vi "Lockin-4461_Multiple Inputs and Outputs_KH_functional_global.vi"(8 "stop":bool) -> ()   [LabVIEW 2013]
uses:
  <vilib>/Analysis/4window.llb/windowTd.ctl
  <vilib>/Analysis/baseanly.llb/Mean (DBL).vi
  <vilib>/Analysis/2dsp.llb/Decimate (single shot, DBL).vi
  <vilib>/DAQmx/write.llb/DAQmx Write (Analog 1D Wfm NChan NSamp).vi
  DAQ-Lockin-SubVI/Lock-in Globles Multiple Inputs and Outputs used with FGV.vi
  <vilib>/DAQmx/miscellaneous.llb/DAQmx Fill In Error Info.vi
  <vilib>/measure/maspectr.llb/FFT Power Spectrum and PSD for N Chan.vi
  <vilib>/Analysis/NI_AALPro.lvlib
  <vilib>/Analysis/NI_AALBase.lvlib
  <vilib>/measure/NI_MAPro.lvlib
panel:
  in  "Input Signals":i16(slide)=2 scale=1.0..20.0
  out "phase log":dbl[](array[numeric])=[0.0, 0.0, 0.0, 0.0, 0.0, 6.661338147750939e-16, 0.0, 1.9984014443252818e-15]
  in  "Tab Control 2":T1(tab)=enum."Lock-in Settings"
  in  "Auto control  max AI rate/ AI block size":bool=TRUE
  in  "AI Buffer Size (S)":i32=10
  in  "AI Block Size":i32=1000
  out "AI Rate":dbl=13000.0 format="%.2f"
  in  "AI Configuration":T2(array[cluster])=[{"AI.Coupling"=10050, "AI.Max"=10.0, "AI.Min"=-10.0, "Input physical channels"="PXI1Slot2/ai0:1"}, {"AI.Coupling"=10050, "AI.Max"=10.0, "AI.Min"=-10.0, "Input physical channels"="PXI1Slot3/ai0:1"}, {"AI.Coupling"=10050, "AI.Max"=10.0, "AI.Min"=-10.0, "Input physical channels"="PXI1Slot5/ai0:1"}, {"AI.Coupling"=10050, "AI.Max"=10.0, "AI.Min"=-10.0, "Input physical channels"="PXI1Slot6/ai0:1"}] {"AI.Coupling" items=["AC"=10045, "DC"=10050, "GND"=10066]}
  in  "AO Configuration":T3(array[cluster])=[{"Output physical channels"="PXI1Slot2/ao0:1", "AO. Max"=0.1, "AO.Min"=-0.1}, {"Output physical channels"="PXI1Slot3/ao0:1", "AO. Max"=0.25, "AO.Min"=-0.25}, {"Output physical channels"="PXI1Slot5/ao0:1", "AO. Max"=0.1, "AO.Min"=-0.1}, {"Output physical channels"="PXI1Slot6/ao0:1", "AO. Max"=0.1, "AO.Min"=-0.1}]
  in  "OSC Configuration":T4(array[cluster])=[[{"Signal Type"=enum."Sine Wave", "DC"=0.0, "Amplitude"=0.01, "frequency"=13.0, "Phase"=0.0}, {"Signal Type"=enum."Sine Wave", "DC"=0.0, "Amplitude"=0.0, "frequency"=13.0, "Phase"=0.0}], [{"Signal Type"=enum."Sine Wave", "DC"=0.0, "Amplitude"=0.0, "frequency"=13.0, "Phase"=0.0}, {"Signal Type"=enum."Sine Wave", "DC"=0.0, "Amplitude"=0.0, "frequency"=13.0, "Phase"=0.0}], [{"Signal Type"=enum."Sine Wave", "DC"=0.0, "Amplitude"=0.0, "frequency"=13.0, "Phase"=0.0}, {"Signal Type"=enum."Sine Wave", "DC"=0.0, "Amplitude"=0.0, "frequency"=13.0, "Phase"=0.0}], [{"Signal Type"=enum."Sine Wave", "DC"=0.0, "Amplitude"=0.0, "frequency"=13.0, "Phase"=0.0}, {"Signal Type"=enum."Sine Wave", "DC"=0.0, "Amplitude"=0.0, "frequency"=13.0, "Phase"=0.0}]] {"frequency" step=0.001 format="%.3p"; "Amplitude" format="%0.2p"; "DC" min=-0.99 max=0.99 format="%.2p"}
  in  "Phase&Tc":T5(array[cluster])=[{"Phase"=0.0, "Time constant"=0.5, "Set Tc"=FALSE, "Autophase"=FALSE, "Order"=0.0}, {"Phase"=0.0, "Time constant"=0.5, "Set Tc"=FALSE, "Autophase"=FALSE, "Order"=0.0}, {"Phase"=0.0, "Time constant"=0.5, "Set Tc"=FALSE, "Autophase"=FALSE, "Order"=0.0}, {"Phase"=0.0, "Time constant"=0.5, "Set Tc"=FALSE, "Autophase"=FALSE, "Order"=0.0}, {"Phase"=0.0, "Time constant"=0.5, "Set Tc"=FALSE, "Autophase"=FALSE, "Order"=0.0}, {"Phase"=0.0, "Time constant"=0.5, "Set Tc"=FALSE, "Autophase"=FALSE, "Order"=0.0}, {"Phase"=0.0, "Time constant"=0.5, "Set Tc"=FALSE, "Autophase"=FALSE, "Order"=0.0}, {"Phase"=0.0, "Time constant"=0.5, "Set Tc"=FALSE, "Autophase"=FALSE, "Order"=0.0}] {"Phase" min=0.0 max=360.0 scale=0.0..360.0}
  in  "Gain":dbl[](array[numeric])=[50000000.0, 50000000.0, 1.0, 1.0, 1.0, 1.0, 1.0, 1.0]
  in  "frequency":dbl=13.0
  out "max ai rate":i32=13000
  out "Numeric":i32=138
  in  "zero offset":bool
  in  "measure offset":bool
  in  "reset lockin & averaging":bool
  out "Display 2":string="-423.350804      n"
  out "Display 1":string="-104.244723      n"
  in  "Remote":bool
  in  "Display":u16(ring) items=["X and Y", "R and Theta"]
  out "Backlog":u8(slide) scale=0.0..100.0
  out "Sampling information":cluster{"Fs":dbl, "#s":dbl}[](array[cluster])=[{"Fs"=13000.0, "#s"=1000.0}]
  out "AO Task":refnum<k21>[](array[refnum])
  out "AI task":refnum<k21>[](array[refnum])
  in  "Tab Control":T6(tab)=enum."Input signals"
  out "Display X (or R) A":dbl[](graph)=[-6.767704118237299e-07, 1.3679095941982762e-06, -8.292119972514093e-07, 1.6081112063430916e-06, -6.48302849428553e-07, 3.3000787620994813e-07, 2.1826626593165523e-07, -4.843594448984296e-07, 7.025229913353154e-07, -4.940803961923873e-07, 5.735003337473624e-07, -3.4668515755027405e-07, -2.4248283537339965e-07, -1.8363287469697745e-08, -3.4589425846339534e-07, 4.6284358832454705e-07, -2.6962179655822256e-07, -1.429402751088828e-07, 9.446578651191532e-08, -5.710117984178673e-09, -5.29242574030563e-07, -7.215176081254315e-08, 2.677231693663559e-07, -2.9474346178622007e-07, 1.6859037233620488e-07, -2.782624102402718e-07, -1.9986912438858682e-07, -3.269593679273288e-08, -2.486510407656373e-07, 5.548402109992747e-07, 9.996987486709427e-08, -6.0130416412624e-08, 9.415818662231201e-08, -2.1083634639079388e-07, 4.091053197976716e-07, -1.1752425483839359e-08, -6.151119173511262e-08, 4.276364767795889e-07, 5.672540816315234e-09, 1.9631938693768442e-07, 3.881923939998436e-07, 3.693414665428258e-07, 2.2443312885204412e-07, -1.0424472343376792e-07, -3.281356459413585e-06, 2.853877661113482e-06, -1.6173510513608656e-06, 2.900242509974247e-07, 3.0449767746807755e-07, -9.53094648189971e-07, 1.19768766975668e-06, -1.6300022513090843e-06, 1.2633381081086798e-06, -1.2597657763077924e-06, 1.5181775758183967e-06, -3.2698180448977813e-07, 4.534684182323745e-22, 2.954958383906869e-22, 2.935987294164666e-22, 2.9919274066034985e-22, 2.4866884846013956e-11, 1.571439962444634e-06, 3.5981993954562916e-05, 4.595320866342681e-05, -3.163614064440566e-05, 2.2025345770237146e-05, -1.4783690228833628e-05, 9.027427496250188e-06, -4.373865947312203e-06, 1.2061179513411652e-06, 2.321934449801555e-06, -3.096117951559957e-06, 3.818767600136303e-06, -2.724223846911526e-06, 2.777457898492608e-06, -1.6318104191727555e-06, 8.644446773102741e-07, 5.245164233996108e-07, -9.074912983112755e-07, 1.5809479476204886e-06, -1.191807434600212e-06, 1.1136104668741203e-06, -8.918436045180084e-07, 7.666775683008394e-07, 4.0094363870758105e-07, -5.024016863890059e-07, 6.184199345905923e-07, -4.547811927193765e-07, 8.577352486006216e-07, -3.929716458984687e-07, -9.250952352542821e-08, 1.4464495001439634e-07, 2.987012020098487e-07, -8.395621078021276e-09, -5.946540278253675e-08, 5.015724336232653e-07, -2.2845172399208505e-07, 2.9148694268542234e-07, -3.3585825169289965e-08, 1.5255809451280384e-07, -1.6688588171069325e-07, 2.9208673634758535e-07, 2.1867560915340566e-08, -1.817033331852077e-09, 2.0922044023006386e-07, -2.0089195447457524e-07, -1.6047621413178067e-07, 3.62693951906398e-07, -4.219972565448854e-07, 2.644775088575862e-07, 1.6782279517097728e-07, -4.0780410649598406e-07, -1.4202551172988562e-07, 4.1098274242707864e-08, 4.0982393853747056e-07, -1.0954576241181e-08, -2.000666884411931e-07, 3.419460779804609e-07, -5.831329333541703e-07, 1.607889368959098e-07, 4.7485928317065607e-07, -1.0986820397700458e-07, 4.234349182513178e-07, 7.50799000900104e-09, -2.913745535551743e-07, 5.212516629832497e-07, -3.5679666811606247e-07, 7.185358920930657e-07, 2.28551626188166e-07, 2.984900132189184e-07, 5.567614355159372e-07, -2.700163649574881e-08, 4.647757728519345e-09, -7.827331963284188e-09, -3.16290394262067e-07, 2.2708072760302243e-07, 7.739366205819891e-08, -4.86859103219973e-07, 2.473259207485168e-07, -3.41601067670072e-07, 1.6627441476941349e-07, 8.910868327391612e-08, -4.126919161116403e-08, 5.064621322918384e-07, -7.216585649893412e-08, 1.7360798289963554e-07, 1.9894946958931327e-07, -1.029870892195247e-07, 1.479174782511515e-08, -7.761128801091328e-08, -9.710807258322806e-08, 2.244692789108791e-07, -5.009546674149695e-07, 2.4630441386600876e-07, 3.701090240857261e-07, -4.940910423104556e-07, 6.97823655978583e-07, 5.463396637012674e-08, 3.3460509656657584e-07, 1.1628795209397034e-07, -9.983904012316269e-08, 2.1194575699660896e-07, -1.4284598126625291e-07, -1.6581535570295627e-07, 1.9543419229659077e-07, 6.421246147653625e-08, 3.817631543808754e-07, 3.5099411367530134e-07, 9.599061510866204e-08, 5.115460403448378e-07, -3.189544820970916e-07, 2.0371122850583007e-07, 7.139469677112191e-08, -2.6780725397357064e-08, 1.8207931762268008e-07, -3.99163483902508e-08, 3.5667336283414435e-24, 2.977721146793187e-22, 2.9488566597725565e-22, 2.931805455672584e-22, 2.8533874679319433e-11, 4.4171853288673887e-07, 1.1776020155369053e-05, 4.5492863810876877e-05, 2.9323742019926304e-05, -2.1525943992685573e-05, 6.085028499678217e-06, 3.4517457636324723e-06, -7.402821485273008e-06, 8.023515280656284e-06, -5.743846711537538e-06, 3.3274091105157146e-06, -7.62703220096605e-07, -1.0696366449954687e-06, 2.5134804524775262e-06, -2.6343637407641244e-06, 2.5318619928474184e-06, -1.7306766758057638e-06, 1.44992950833644e-06, 1.4483945167047895e-07]
  out "Display Y (or Theta) A":dbl[](graph)=[4.765499299686936e-07, -9.658586916637982e-07, -7.621778309143253e-08, -1.5258147249425879e-07, -2.4990753387284357e-07, 1.3419411932204113e-07, -8.565299692875945e-07, 5.571108791407577e-07, -7.860547079397809e-08, -7.196286228942718e-07, 3.4315278763967647e-07, -6.204384175643328e-07, 1.774316085303007e-07, 1.375503590545208e-07, -9.027207823009459e-07, 4.7108028753992357e-07, -1.4273262355224388e-07, -5.084378639622054e-07, 2.0064639544519283e-07, -6.100241361118937e-07, 3.5508186140312606e-07, 1.6599492404614552e-07, -1.1241242632694126e-06, 3.545737663988187e-07, -1.3680834360003273e-07, -5.671646797482132e-07, 3.003111466009731e-07, -7.790822713575479e-07, 3.293880422749827e-07, 3.28274379240407e-08, -1.0651740914596076e-06, 4.2770794764999845e-07, -5.104224380786051e-07, -2.472151922016114e-07, 1.9800282516829894e-07, -7.284254119168647e-07, 5.863115303219669e-07, -2.81773970579004e-07, -7.156335675351997e-07, 2.3981773570157667e-07, -3.978801443495009e-07, 3.035512690481674e-07, -1.7158995838277135e-07, -4.233508035480193e-07, -8.088850970477616e-07, 6.737027936126898e-07, -1.759072178658265e-07, -6.972834404887968e-07, 1.272488135816818e-06, -1.2086621076536852e-06, 4.69525474705048e-07, -4.919175010780031e-08, -3.50864282590232e-07, 6.020350472256037e-07, -9.484640076506137e-07, -6.830224693863262e-08, 1.0170935534147539e-22, -8.29623972830081e-22, -8.014563293027786e-22, -8.094000243152346e-22, 1.3353078985706605e-11, 1.6373548472325611e-07, 1.4866311767580978e-06, -2.707411790797605e-06, 6.830995141435044e-07, -3.8763934216822793e-07, -3.894235373830128e-07, -9.303274404957174e-08, -1.5541472171160917e-07, -1.0548850159824638e-06, 1.301686262269789e-06, -1.9557074574821375e-06, 9.368644690210887e-07, -5.392324932206546e-07, -1.0317815283114626e-06, 9.503284335604831e-07, -1.1138402195810916e-06, -8.612001299094237e-08, 3.392287632745269e-07, -9.880574731396456e-07, 6.176942647460194e-07, -5.670403477561947e-07, -7.529082791811021e-08, 3.797538713075729e-07, -6.875418705429333e-07, 3.774689030428864e-08, 4.010310610815791e-07, -5.552428738314573e-07, 3.8499536868861883e-07, -6.445873434134007e-07, -3.326615731244241e-07, 4.502182873700019e-07, -7.750874192225206e-07, 4.117923202917222e-07, -6.431352998299419e-07, 3.5044644716276235e-07, -1.4225277208615523e-07, -6.876478797176894e-07, 5.399420578514256e-07, -4.5606838526251626e-07, -1.2810883746936567e-07, 7.507205080273586e-07, -1.4012460201934012e-06, 3.6687827494239255e-07, -2.4916075902104696e-07, -6.048091008906423e-07, 6.617540494081048e-07, -1.017139965154715e-06, 6.302573641557335e-07, 4.555496901851896e-07, -1.3339391648309178e-06, 6.715666266662573e-07, -3.8798990954152797e-07, -3.6012440675569084e-07, 5.414910168700109e-07, -1.3243576755919245e-06, 5.902559482413635e-07, -7.542190392147796e-08, -1.0785352133753382e-06, 9.869413956855774e-07, -9.442478036537707e-07, -4.8555902344221593e-08, 5.874045024703844e-07, -1.1585692990263365e-06, 1.3486079750496373e-06, -5.071584526584705e-07, -5.100916917445276e-07, 6.330937674492109e-07, -1.235592399497452e-06, 9.223862720486185e-07, 6.04251856246877e-08, -1.2764854943402043e-06, 8.83547168218078e-07, -9.047288617993288e-07, 2.0116909352114474e-07, 5.358138396845644e-07, -1.3168565866224215e-06, 4.095307061714363e-07, -6.27867381040266e-07, -4.472555022141913e-07, 8.124683056348434e-07, -6.96815296189946e-07, -1.3075261738966236e-07, -2.448175089906454e-07, -3.31091978464826e-07, 4.938406467055916e-07, -1.0121928097926847e-06, 2.6683471402237015e-07, -3.854622779756573e-07, -6.116229848120615e-07, 7.413846592203119e-07, -3.878576789341664e-07, -4.803212369821987e-09, -1.512740254582647e-07, -9.37733298786493e-07, 3.083451264193004e-07, -7.278473080315107e-07, -2.1621978373244913e-07, 1.1649243053043013e-06, -1.5574296555740364e-06, 2.0216029416288657e-07, -1.738290377715283e-08, -8.124252331847678e-07, 8.556517228357048e-07, -1.1895268912765046e-06, -1.6299284686030149e-07, 5.025591222770188e-07, -1.256876728303257e-06, 4.966801881381768e-07, -2.653578297740131e-07, -7.841925208481243e-07, 6.961355949365849e-07, -1.3545884441334733e-06, 1.8978106285789698e-07, -3.1292466455277164e-07, -1.116079741754174e-06, 6.606025379921262e-24, -7.987352443116322e-22, -8.305769155450611e-22, -8.014315043874178e-22, 1.528632786785048e-11, 5.851716352372578e-08, 7.012774926585611e-07, 7.260202605191567e-07, -1.8385722657507987e-06, -7.48491270371179e-07, 1.078630704871155e-06, -5.895807456908318e-07, 1.4658536078852006e-07, 1.0975439156015532e-07, -4.165723785464372e-07, -6.413089995227893e-08, 2.3302809137460278e-07, -4.5082625792713e-08, 1.8812524970362413e-07, 1.2661990176118822e-08, -9.607065782256097e-07, 4.267709983481109e-07, -7.948677906464168e-08, -2.6388811975329723e-07]
  out "Waveform Graph":waveform(dbl)[](graph)=[{"t0"=timestamp(3506383757.1591763 s since 1904-01-01), "dt"=7.692307684820771e-05, "Y"=array[1000 elements], "attributes"=variant("NI_ChannelName"=variant(string "PXI1Slot2/ai0"), "NI_UnitDescription"=variant(string "Volts"))}, {"t0"=timestamp(3506383757.1591763 s since 1904-01-01), "dt"=7.692307684820771e-05, "Y"=array[1000 elements], "attributes"=variant("NI_ChannelName"=variant(string "PXI1Slot2/ai1"), "NI_UnitDescription"=variant(string "Volts"))}, {"t0"=timestamp(3506383757.1600227 s since 1904-01-01), "dt"=7.692307684820771e-05, "Y"=array[1000 elements], "attributes"=variant("NI_ChannelName"=variant(string "PXI1Slot3/ai0"), "NI_UnitDescription"=variant(string "Volts"))}, {"t0"=timestamp(3506383757.1600227 s since 1904-01-01), "dt"=7.692307684820771e-05, "Y"=array[1000 elements], "attributes"=variant("NI_ChannelName"=variant(string "PXI1Slot3/ai1"), "NI_UnitDescription"=variant(string "Volts"))}, {"t0"=timestamp(3506383757.1600227 s since 1904-01-01), "dt"=7.692307684820771e-05, "Y"=array[1000 elements], "attributes"=variant("NI_ChannelName"=variant(string "PXI1Slot5/ai0"), "NI_UnitDescription"=variant(string "Volts"))}, {"t0"=timestamp(3506383757.1600227 s since 1904-01-01), "dt"=7.692307684820771e-05, "Y"=array[1000 elements], "attributes"=variant("NI_ChannelName"=variant(string "PXI1Slot5/ai1"), "NI_UnitDescription"=variant(string "Volts"))}, {"t0"=timestamp(3506383757.1600227 s since 1904-01-01), "dt"=7.692307684820771e-05, "Y"=array[1000 elements], "attributes"=variant("NI_ChannelName"=variant(string "PXI1Slot6/ai0"), "NI_UnitDescription"=variant(string "Volts"))}, {"t0"=timestamp(3506383757.1600227 s since 1904-01-01), "dt"=7.692307684820771e-05, "Y"=array[1000 elements], "attributes"=variant("NI_ChannelName"=variant(string "PXI1Slot6/ai1"), "NI_UnitDescription"=variant(string "Volts"))}]
  in  "Stream to disk?":bool
  in  "decimating factor":i32
  in  "decimating factor 2":i32=1
  out "Waveform Graph 2":cluster{"f0":dbl, "df":dbl, "magnitude":dbl[]}[](graph)
  in  "window":T7=1 items=["Rectangle"=0, "Hanning"=1, "Hamming"=2, "Blackman-Harris"=3, "Exact Blackman"=4, "Blackman"=5, "Flat Top"=6, "4 Term B-Harris "=7, "7 Term B-Harris"=8, "Low Sidelobe"=9, "Blackman Nuttall"=11, "Triangle"=30, "Bartlett-Hanning"=31, "Bohman"=32, "Parzen"=33, "Welch"=34, "Kaiser"=60, "Dolph-Chebyshev"=61, "Gaussian"=62]
  in  "averaging parameters":T8={"averaging mode"=enum."No averaging", "weighting mode"=enum."Exponential", "number of averages"=10} {"number of averages" min=1}
  in  "dB On (F)":bool
  in  "Rolling Avg Parameters":T9={"Rolling Avg mode"=enum."No Averaging", "# of averages"=10} {"# of averages" min=1}
  in  "Filter Type":T10(ring)=enum."Chebyshev"
  in  "Cutoff Freq":dbl[unit]=0.9 format="%.2f"
  out "Results (X, Y, R, Theta)":dbl[][](array[numeric])=[[-8.990938951699043e-08, -5.496874633933286e-07, 5.569919260950825e-07, -99.28930194172699], [-1.0424472343376792e-07, -4.233508035480193e-07, 4.3599640506377615e-07, -103.83315475232594], [-8.663279130692378e-08, -2.555950511771059e-07, 2.6987788111636043e-07, -108.72385784210852], [-3.572835649086049e-08, -7.56786271488616e-08, 8.368853006639814e-08, -115.2722910768039], [4.431812686724637e-08, 8.517364090161592e-08, 9.601377751895176e-08, 62.51083208252897], [1.4523643643592666e-07, 1.9896598237318188e-07, 2.4633530930488284e-07, 53.87219602328508]] format="%#_6p"
  out "Measure?":u16[](array[numeric])
  in  "Cluster (unused right now)":T11={"Amplitude"=[0.001, 2e-08, 0.001, 0.001, 0.001, 2e-08], "DC"=[0.001, 2e-08, 0.001, 0.001, 0.001, 2e-08], "phase"=[0.001, 2e-08, 0.001, 0.001, 0.001, 2e-08], "Array"=[]}
  out "offsets":dbl[](array[numeric])
  # "*****Customized for 4461 + 4462 cards; functional globals*****"
  # "Real time Adjustable Values"
  # "Configurations"
  # "should this be x multiple\nof the frequency?"
  # "The top array index selects which card you are setting the outputs for,and the second index selects which output chanel on that card.\n\nFor Phase&Tc, you must have an array element initialized for each input signal."
  # "Features:\n1, Any number of input and output channels\n2, Each AO outputs an DC+AC signal, DC for sample biasing and AC for OSC. These values can be adjusted in real time.\n3, Synchronous filtering\n\nInstructions:\n1, Array index of AI configuration and AO configuration refers to task.\n2, Array index in Amplifier Settings, Phase$&Tc control , and gains correlates to channel number.\n3, Each 4461 board can have 2 lock-in channels. Syntax for 2 channles, e.g. PXI1Slot2/ai0:1. If you want to use just one, then PXI1Slot2/ai0.\n4, Parameters (especially DC value for sample biasing) can be remotely controlled by clicking \"local\"and \"remote\" button. In real experiments, put golable values (can be found in Lock-in globles.vi) in your VI to control the lock-in and read out.\n5, choose OSC frequencies to be multiple of \nAI Rate/AI Block SIze to have best performance.\n\n-Guanglei 06/23/2011\n\nUpdate:\n1. Allows any number of lockin amplifiers and AO tasks.\n2. Delete the channels from any AI/AO Configuration elements you do not want to use.\n3. Rows (first index) of the OSC Configuration correspond to different AO tasks, while columns (second index) correspond to AO channels in that task. All channels in a given element of the AO Configuration array will go into a single task.\n4. The same number of output channels must go in each AO task.\n5. Make sure a Phase&Tc element and an Amplifier Settings element is set for each AI channel.\n-Joe 12/3/2013"
  # "hide stuff here in this tab"
  # "multiple of frequency??"
  # "this is \"time constant\""
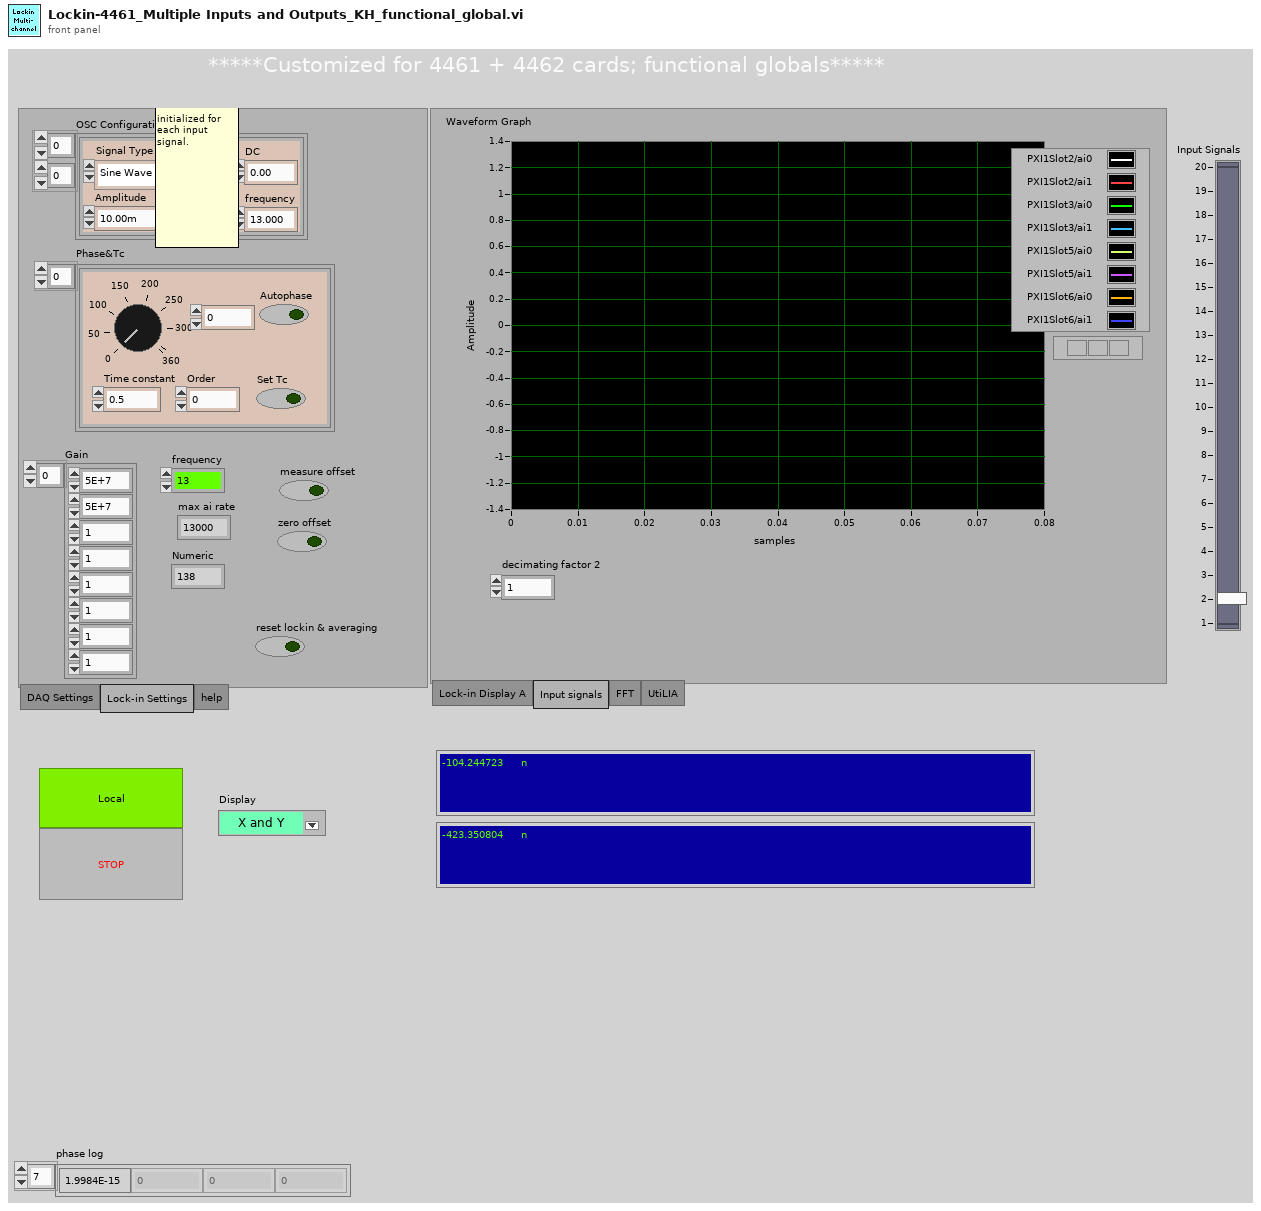
[diagram p1: front panel]
types:
  T1 = enum32{"DAQ Settings", "Lock-in Settings", "help"}
  T2 = cluster{"AI.Coupling":i32, "AI.Max":dbl, "AI.Min":dbl, "Input physical channels":tag}[]
  T3 = cluster{"Output physical channels":tag, "AO. Max":dbl, "AO.Min":dbl}[]
  T4 = cluster{"Signal Type":enum16{"Sine Wave", "Triangle Wave", "Square Wave", "Sawtooth Wave"}, "DC":dbl, "Amplitude":dbl, "frequency":dbl, "Phase":dbl}[][]
  T5 = cluster{"Phase":dbl, "Time constant":dbl, "Set Tc":bool, "Autophase":bool, "Order":dbl}[]
  T6 = enum32{"Lock-in Display A", "Input signals", "FFT", "UtiLIA"}
  T7 = typedef "NI_AALPro.lvlib/windowTd.ctl" = u32
  T8 = cluster{"averaging mode":enum16{"No averaging", "Vector averaging", "RMS averaging", "Peak hold"}, "weighting mode":enum16{"Linear", "Exponential"}, "number of averages":u32}
  T9 = cluster{"Rolling Avg mode":enum16{"No Averaging", "Linear", "Exponential"}, "# of averages":u32}
  T10 = enum16{"None", "Butterworth", "Chebyshev", "Inv Chebyshev"}
  T11 = cluster{"Amplitude":dbl[], "DC":dbl[], "phase":dbl[], "Array":enum16{"Sine Wave", "Triangle Wave", "Square Wave", "Sawtooth Wave"}[]}
  T12 = cluster{"Signal Type":enum16{"Sine Wave", "Triangle Wave", "Square Wave", "Sawtooth Wave"}, "DC":dbl, "Amplitude":dbl, "frequency":dbl, "Phase":dbl}
  T13 = cluster{"Ref X":dbl[], "Ref Y":dbl[], "AI Rate":dbl, "AI Block Size":dbl, "Frequency":dbl, "Ref amp":dbl}[]
  T14 = cluster{"Ref X":dbl[], "Ref Y":dbl[], "AI Rate":dbl, "AI Block Size":dbl, "Frequency":dbl, "Ref amp":dbl}
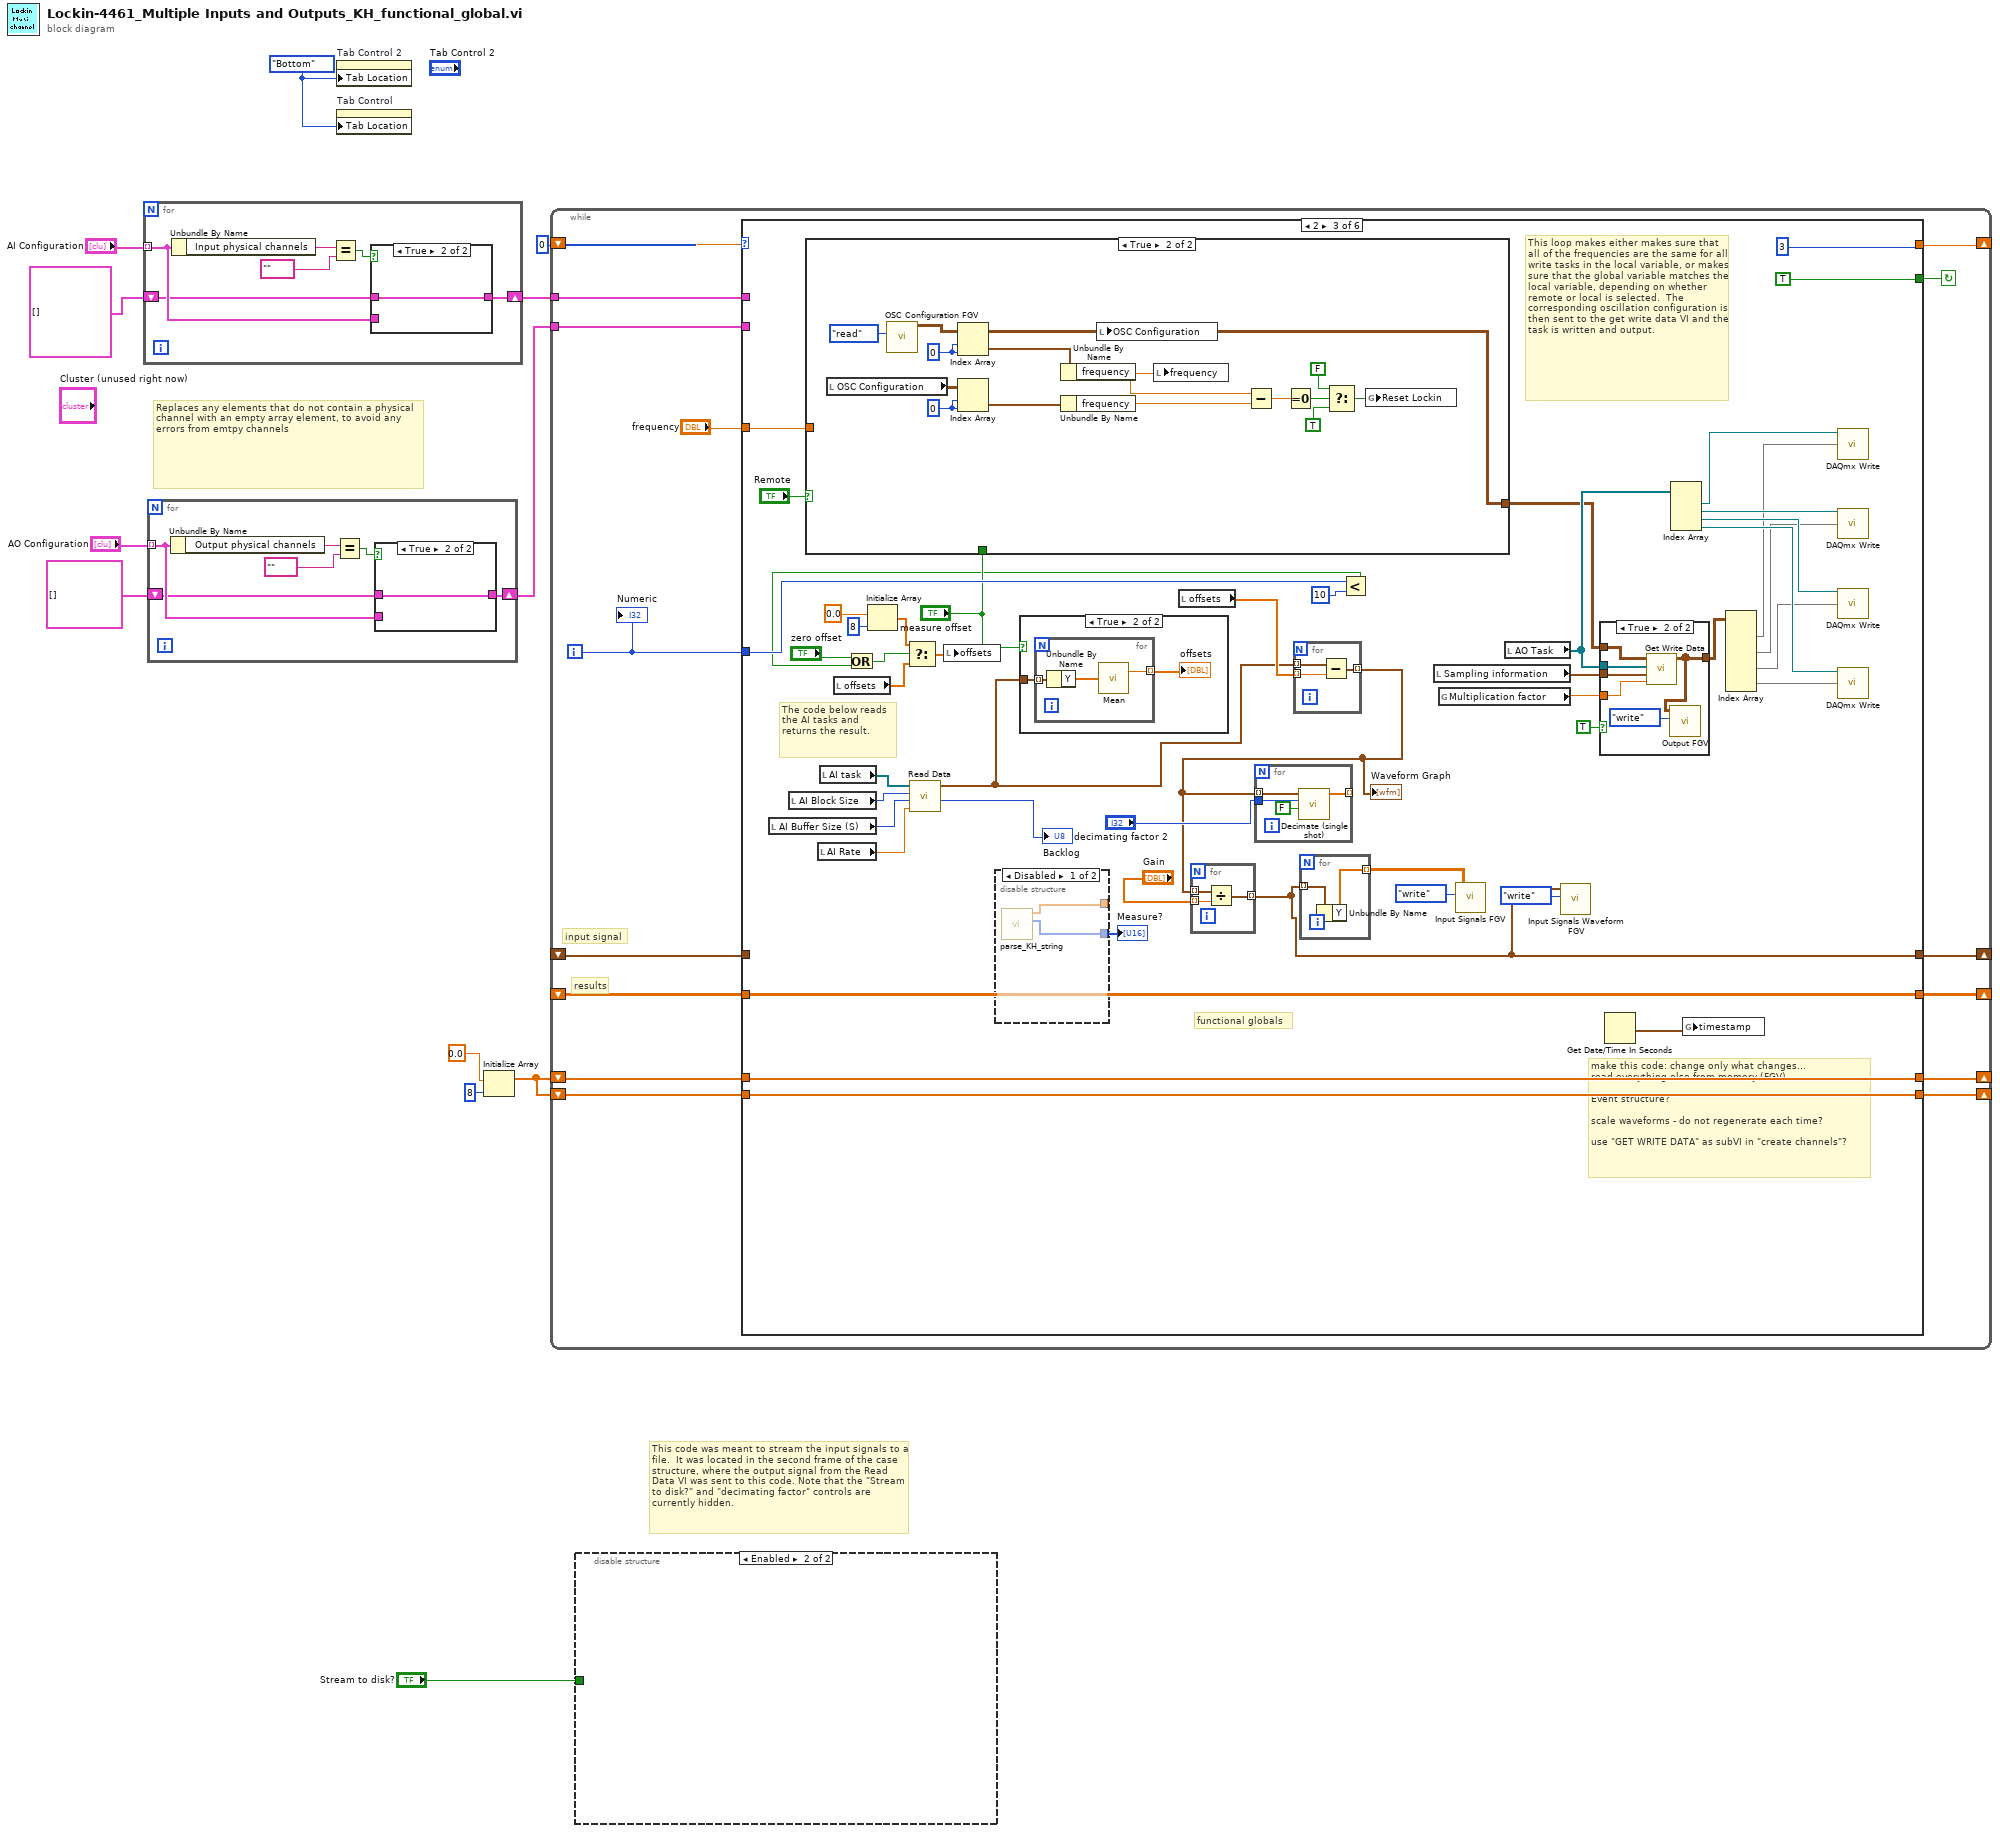
[diagram p0: block diagram]
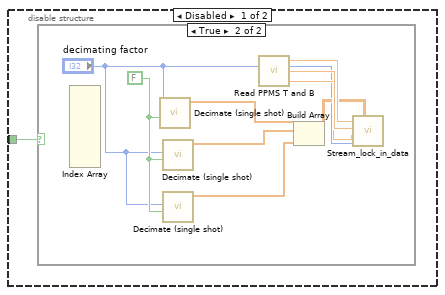
[diagram p2: hidden frame]
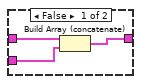
[diagram p4: hidden frame]
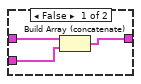
[diagram p5: hidden frame]
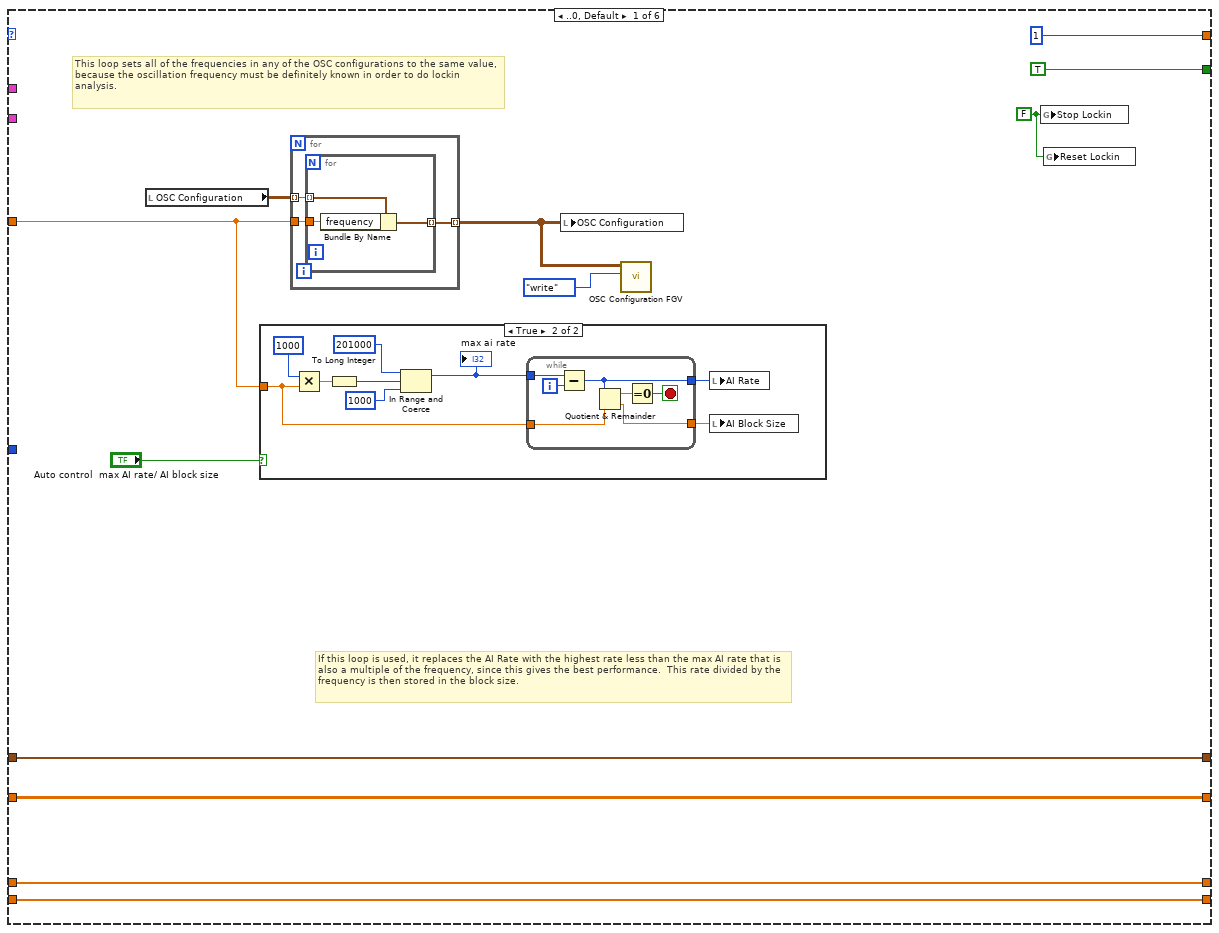
[diagram p6: hidden frame]
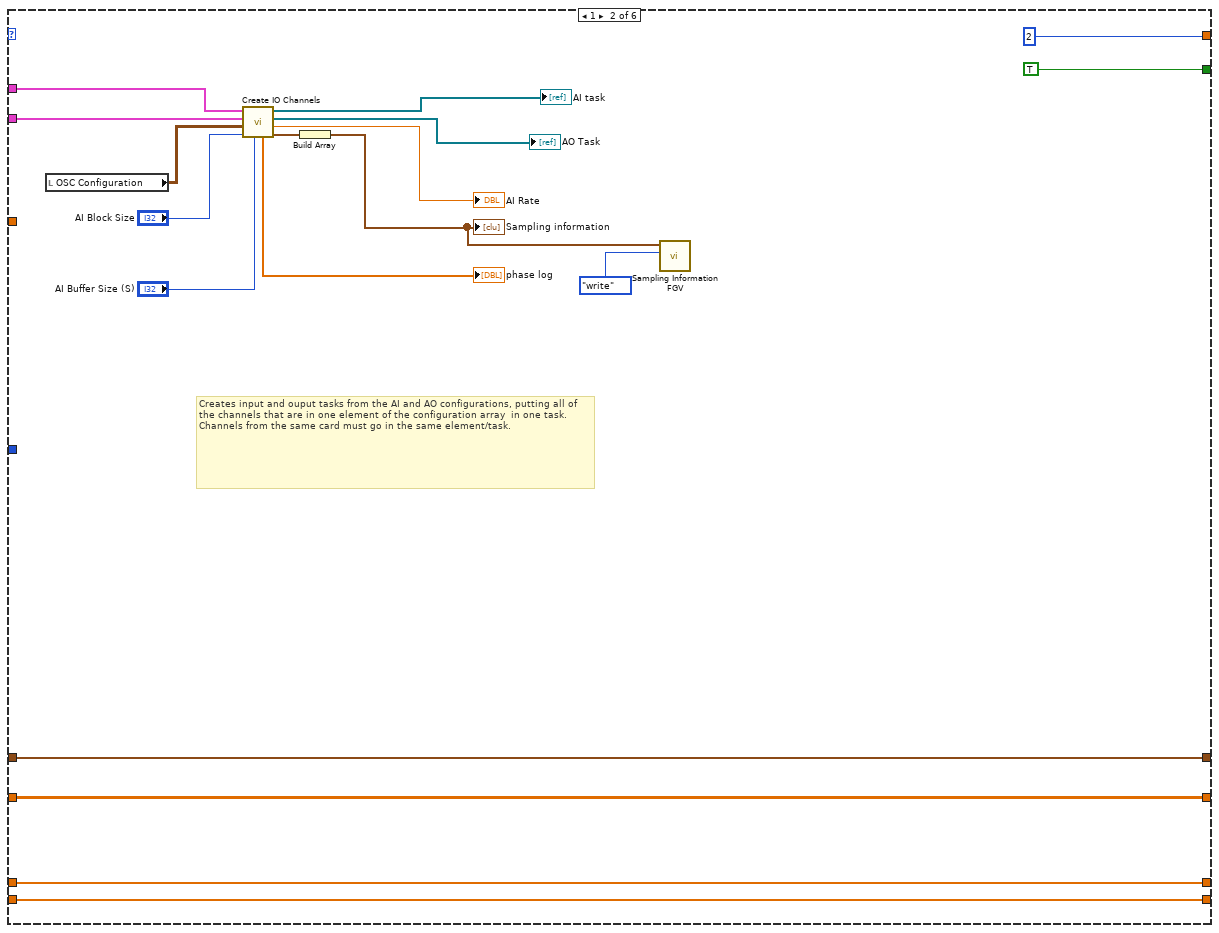
[diagram p8: hidden frame]
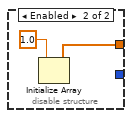
[diagram p10: hidden frame]
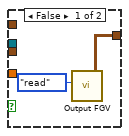
[diagram p11: hidden frame]
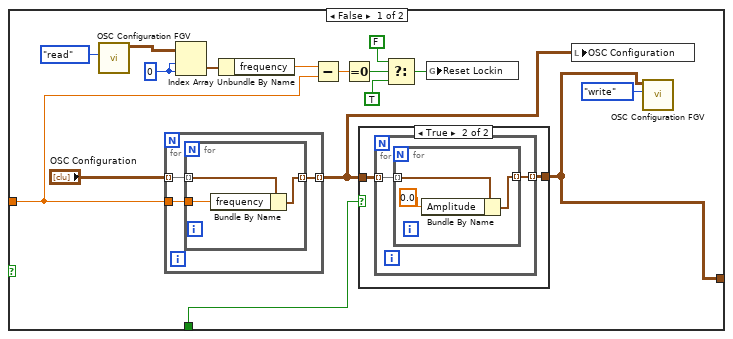
[diagram p12: hidden frame]
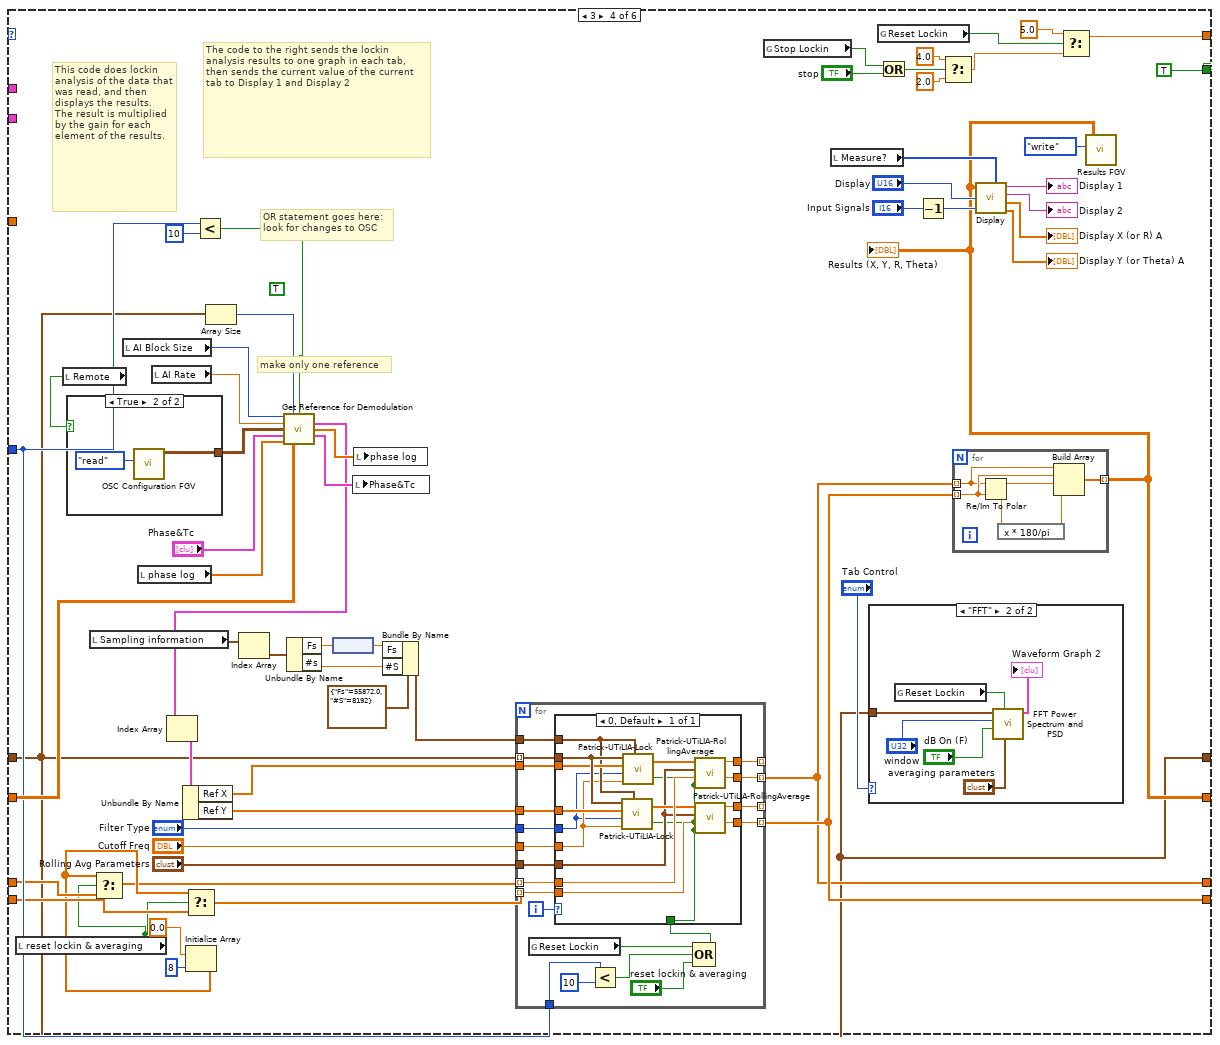
[diagram p14: hidden frame]
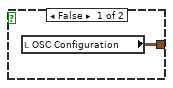
[diagram p16: hidden frame]
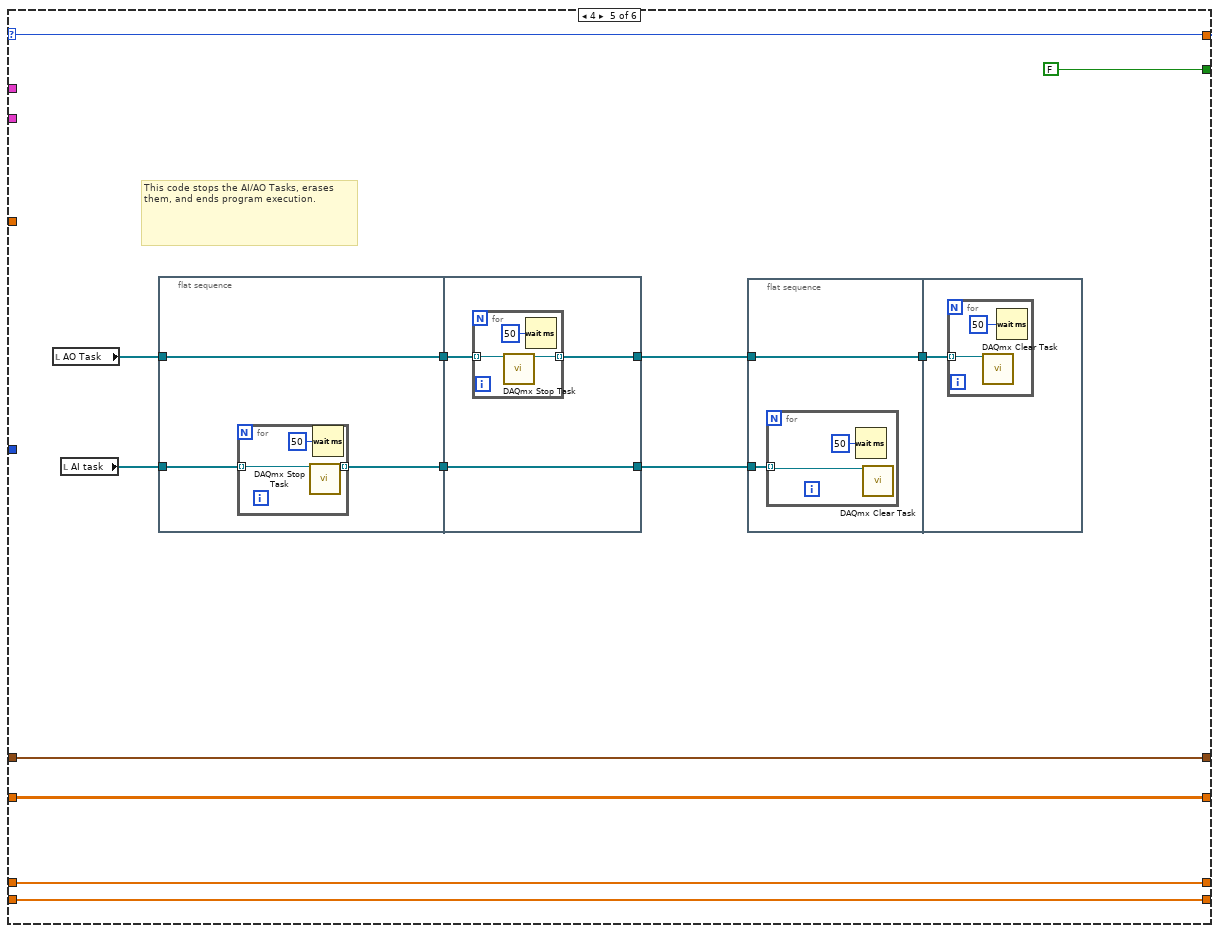
[diagram p17: hidden frame]
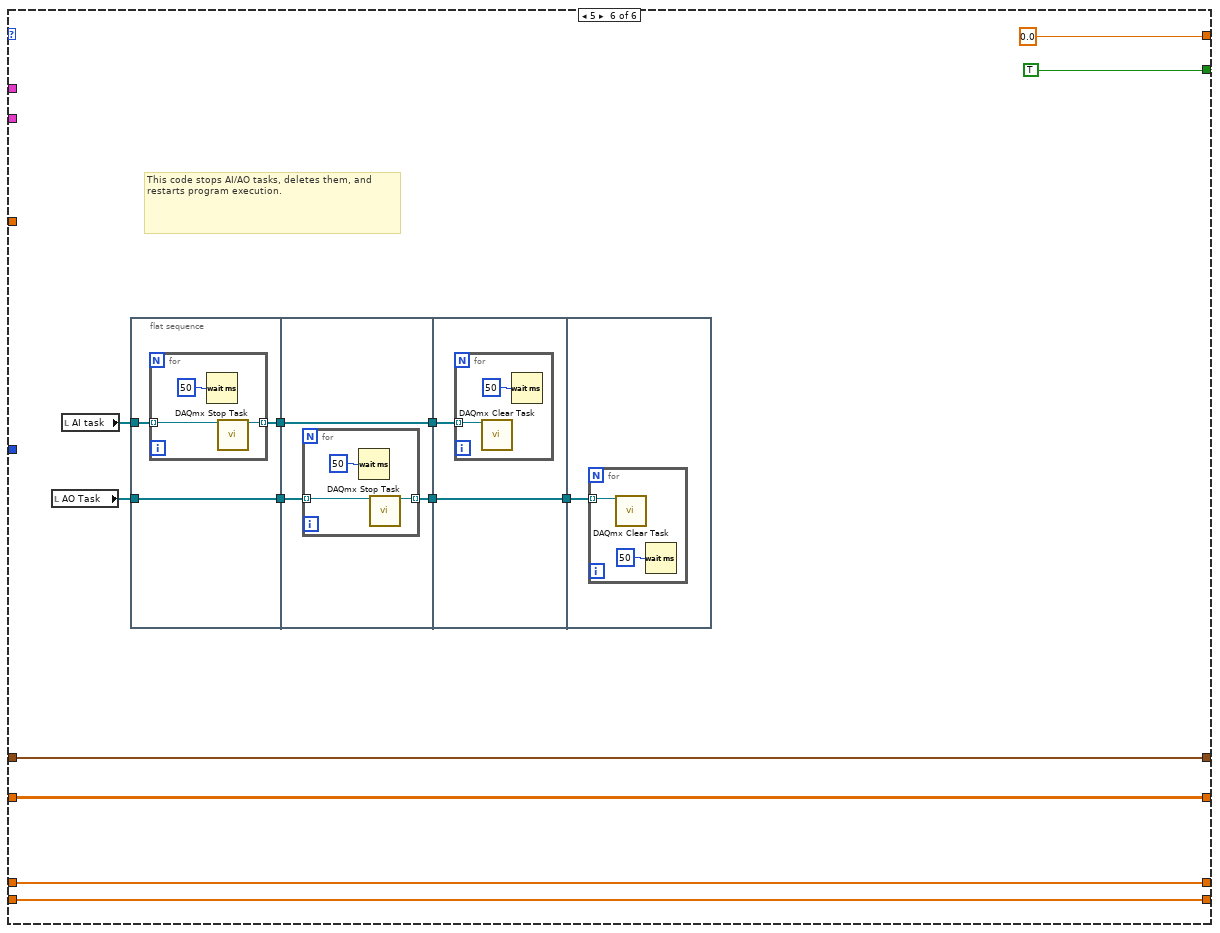
[diagram p18: hidden frame]
diagram:
  w6 = enum32{"Top", "Bottom", "Left", "Right"}."Bottom" ("Tab Location")
  # "This code was meant to stream the input signals to a file.  It was located in the second frame of the case structure, where the output signal from the Read Data VI was sent to this code. Note that the \"Stream to disk?\" and \"decimating factor\" controls are currently hidden."
  # "Replaces any elements that do not contain a physical channel with an empty array element, to avoid any errors from emtpy channels"
  n1 = for {
    tunnel: "AI Configuration" -> [w15] mode=indexing
    shift-right: [w13] -> w12
    shift-left: T2 [] ("AI Configuration") -> [w14]
    n2 = Unbundle By Name(w15) -> ("Input physical channels"=w17:tag)
    n3 = Equal?(x=w17, y=tag "" ("Empty physical channels")) -> (x = y?=w18:bool)
    n4 = case shown="True" w18 {
      tunnel: w15 -> [w20 _]
      tunnel: w14 -> [w21 w22]
      tunnel: [w19 w22] -> w13
      frame False {
        n5 = Build Array (concatenate)(w21, w20) -> (w19:T2)
      }
      frame True {
      }
    }
  }
  n6 = for {
    tunnel: "AO Configuration" -> [w25] mode=indexing
    shift-right: [w23] -> w4
    shift-left: T3 [] ("AO Configuration 2") -> [w24]
    n7 = Unbundle By Name(w25) -> ("Output physical channels"=w27:tag)
    n8 = Equal?(x=w27, y=tag "" ("Empty physical channels")) -> (x = y?=w28:bool)
    n9 = case shown="True" w28 {
      tunnel: w25 -> [w30 _]
      tunnel: w24 -> [w31 w32]
      tunnel: [w29 w32] -> w23
      frame False {
        n10 = Build Array (concatenate)(w31, w30) -> (w29:T3)
      }
      frame True {
      }
    }
  }
  n11 = property on="Tab Control 2" class="TabCtl (strict)"("Tab Location"=w6) -> ()  [unwired: 2 in, 2 out]
  n12 = property on="Tab Control" class="TabCtl (strict)"("Tab Location"=w6) -> ()  [unwired: 2 in, 2 out]
  n13 = Initialize Array(0.0, 8 ("dimension size")) -> (w2:dbl[])
  n14 = while {
    shift-right: [w47] -> _
    shift-left: 0 -> [w46]
    tunnel: w12 -> [w45]
    tunnel: w4 -> [w43]
    shift-right: [w42] -> _
    shift-left: _ -> [w41]
    shift-right: [w39] -> _
    shift-left: _ -> [w40]
    shift-right: [w36] -> _
    shift-left: w2 -> [w34]
    shift-right: [w37] -> _
    shift-left: w2 -> [w35]
    i -> [w38]
    stop <- w44 continue-if-true
    # "results"
    # "input signal"
    n15 = case shown="2" w46 {
      selector: w46 -> [_ _ _ _ w342 _]
      tunnel: [1 2 3 w271 w342 0.0 ("f")] -> w47
      tunnel: w45 -> [_ w94 _ _ _ _]
      tunnel: [TRUE TRUE TRUE TRUE FALSE TRUE] -> w44
      tunnel: w43 -> [_ w93 _ _ _ _]
      tunnel: [w52 w88 w102 w222 w334 w366] -> w42
      tunnel: w41 -> [w52 w88 _ w222 w334 w366]
      tunnel: w40 -> [w51 w87 w125 w251 w333 w365]
      tunnel: [w51 w87 w125 w224 w333 w365] -> w39
      tunnel: w38 -> [_ _ w115 w241 _ _]
      tunnel: [w50 w84 w121 w235 w332 w364] -> w37
      tunnel: [w49 w83 w120 w234 w331 w363] -> w36
      tunnel: w35 -> [w50 w84 w121 w230 w332 w364]
      tunnel: w34 -> [w49 w83 w120 w229 w331 w363]
      tunnel: "frequency" -> [w48 _ w119 _ _ _]
      frame ..0, Default {
        w58 = FALSE ("Stop Lockin")
        # "If this loop is used, it replaces the AI Rate with the highest rate less than the max AI rate that is also a multiple of the frequency, since this gives the best performance.  This rate divided by the frequency is then stored in the block size."
        # "This loop sets all of the frequencies in any of the OSC configurations to the same value, because the oscillation frequency must be definitely known in order to do lockin analysis."
        n16 = local read "OSC Configuration"() -> (w55:T4)
        n17 = case shown="True" "Auto control  max AI rate/ AI block size" {
          tunnel: w48 -> [_ w66]
          frame False {
          }
          frame True {
            n18 = Multiply(x=1000, y=w66) -> (x*y=w72:dbl)
            n19 = To Long Integer(number=w72) -> (32bit integer=w70:i32)
            n20 = In Range and Coerce(upper limit=201000, x=w70, lower limit=1000) -> (coerced(x)=w67:i32)  [unwired: 1 out]
            "max ai rate" <- w67
            n21 = while {
              tunnel: w67 -> [w81]
              tunnel: [w79] -> w74
              tunnel: [w77] -> w73
              tunnel: w66 -> [w78]
              i -> [w80]
              stop <- w75 stop-if-true
              n22 = Subtract(x=w81, y=w80) -> (x-y=w77:i32)
              n23 = Quotient & Remainder(x=w77, y=w78) -> (x-y*floor(x/y)=w76:dbl, floor(x/y)=w79:dbl)
              n24 = Equal To 0?(x=w76) -> (x = 0?=w75:bool)
            }
            n25 = local write "AI Rate"(w73) -> ()
            n26 = local write "AI Block Size"(w74) -> ()
          }
        }
        n27 = for {
          tunnel: w55 -> [w62] mode=indexing
          tunnel: [w61] -> w54 mode=indexing
          tunnel: w48 -> [w60]
          n28 = for {
            tunnel: w62 -> [w65] mode=indexing
            tunnel: [w64] -> w61 mode=indexing
            tunnel: w60 -> [w63]
            n29 = Bundle By Name(cluster=w65, "frequency"=w63) -> (w64:T12)
          }
        }
        n30 = local write "OSC Configuration"(w54) -> ()
        n31 = call "OSC Configuration FGV.vi"("Function"=enum16{"write", "read"}."write", "OSC Configuration"=w54) -> ()  [unwired: 4 in, 2 out]
        n32 = global write "Lock-in Globles Multiple Inputs and Outputs used with FGV.vi" "Stop Lockin"(w58) -> ()
        n33 = global write "Lock-in Globles Multiple Inputs and Outputs used with FGV.vi" "Reset Lockin"(w58) -> ()
      }
      frame 1 {
        # "Creates input and ouput tasks from the AI and AO configurations, putting all of the channels that are in one element of the configuration array  in one task.  Channels from the same card must go in the same element/task."
        n34 = local read "OSC Configuration"() -> (w97:T4)
        n35 = call "Create IO Channels.vi"("AI Buffer Size (s)"="AI Buffer Size (S)", "AI Block Size"="AI Block Size", "OSC Configuration"=w97, "AO Configuration"=w93, "AI Configuration"=w94) -> ("sampling info"=w89:cluster{"Fs":dbl, "#s":dbl}, "AI Rate"=→"AI Rate":dbl, "AO Task"=→"AO Task":refnum<k21>[], "AI task"=→"AI task":refnum<k21>[], "phase log"=→"phase log":dbl[])  [unwired: 1 in, 1 out]
        n36 = Build Array(w89) -> (w82:cluster{"Fs":dbl, "#s":dbl}[])
        "Sampling information" <- w82
        n37 = call "Sampling Information FGV.vi"("Function"=enum16{"write", "read"}."write", "Sampling information"=w82) -> ()  [unwired: 4 in, 2 out]
      }
      frame 2 {
        # "make this code: change only what changes...\nread everything else from memory (FGV)\n\nEvent structure?\n\nscale waveforms - do not regenerate each time?\n\nuse \"GET WRITE DATA\" as subVI in \"create channels\"?"
        # "functional globals"
        # "The code below reads the AI tasks and returns the result."
        # "This loop makes either makes sure that all of the frequencies are the same for all write tasks in the local variable, or makes sure that the global variable matches the local variable, depending on whether remote or local is selected.  The corresponding oscillation configuration is then sent to the get write data VI and the task is written and output."
        n38 = local read "AI Buffer Size (S)"() -> (w139:i32)
        n39 = local read "AI Block Size"() -> (w140:i32)
        n40 = case shown="True" "Remote" {
          tunnel: [w177 w207] -> w124
          tunnel: w119 -> [w180 _]
          tunnel: "measure offset" -> [w179 _]
          frame False {
            w189 = 0 ("index")
            n41 = call "OSC Configuration FGV.vi"("Function"=enum16{"write", "read"}."read") -> ("OSC Configuration"=w183:T4)  [unwired: 5 in, 1 out]
            n42 = for {
              tunnel: w180 -> [w203]
              tunnel: "OSC Configuration" -> [w202] mode=indexing
              tunnel: [w201] -> w178 mode=indexing
              n43 = for {
                tunnel: w202 -> [w206] mode=indexing
                tunnel: w203 -> [w205]
                tunnel: [w204] -> w201 mode=indexing
                n44 = Bundle By Name(cluster=w206, "frequency"=w205) -> (w204:T12)
              }
            }
            n45 = Index Array(array=w183, index (row)=w189, index (col)=w189) -> (element=w188:T12)
            n46 = Unbundle By Name(w188) -> ("frequency"=w182:dbl)
            n47 = Subtract(x=w182, y=w180) -> (x-y=w181:dbl)
            n48 = Equal To 0?(x=w181) -> (x = 0?=w187:bool)
            n49 = case shown="True" w179 {
              tunnel: w178 -> [w193 w195]
              tunnel: [w193 w194] -> w177
              frame False {
              }
              frame True {
                n50 = for {
                  tunnel: w195 -> [w197] mode=indexing
                  tunnel: [w196] -> w194 mode=indexing
                  n51 = for {
                    tunnel: w197 -> [w200] mode=indexing
                    tunnel: [w199] -> w196 mode=indexing
                    n52 = Bundle By Name(cluster=w200, "Amplitude"=0.0) -> (w199:T12)
                  }
                }
              }
            }
            n53 = Select(t=FALSE ("Reset Lockin"), s=w187, f=TRUE ("Reset Lockin")) -> (s? t:f=w184:bool)
            n54 = global write "Lock-in Globles Multiple Inputs and Outputs used with FGV.vi" "Reset Lockin"(w184) -> ()
            n55 = local write "OSC Configuration"(w178) -> ()
            n56 = call "OSC Configuration FGV.vi"("Function"=enum16{"write", "read"}."write", "OSC Configuration"=w177) -> ()  [unwired: 4 in, 2 out]
          }
          frame True {
            w217 = 0 ("index")
            w219 = 0 ("index")
            n57 = local read "OSC Configuration"() -> (w209:T4)
            n58 = call "OSC Configuration FGV.vi"("Function"=enum16{"write", "read"}."read") -> ("OSC Configuration"=w207:T4)  [unwired: 5 in, 1 out]
            n59 = Index Array(array=w207, index (row)=w219, index (col)=w219) -> (element=w220:T12)
            n60 = Index Array(array=w209, index (row)=w217, index (col)=w217) -> (element=w216:T12)
            n61 = Unbundle By Name(w220) -> ("frequency"=w208:dbl)
            n62 = Unbundle By Name(w216) -> ("frequency"=w214:dbl)
            n63 = local write "OSC Configuration"(w207) -> ()
            n64 = local write "frequency"(w208) -> ()
            n65 = Subtract(x=w208, y=w214) -> (x-y=w215:dbl)
            n66 = Equal To 0?(x=w215) -> (x = 0?=w213:bool)
            n67 = Select(t=FALSE ("Reset Lockin"), s=w213, f=TRUE ("Reset Lockin")) -> (s? t:f=w210:bool)
            n68 = global write "Lock-in Globles Multiple Inputs and Outputs used with FGV.vi" "Reset Lockin"(w210) -> ()
          }
        }
        n69 = local read "AI Rate"() -> (w138:dbl)
        n70 = local read "AI task"() -> (w141:refnum<k21>[])
        n71 = local read "offsets"() -> (w113:dbl[])
        n72 = Initialize Array(0.0, 8 ("dimension size")) -> (w110:dbl[])
        n73 = call "Read Data.vi"("AI Rate"=w138, "AI Buffer Size (s)"=w139, "AI Block Size"=w140, "AI task"=w141) -> ("Backlog"=→"Backlog":u8, "Input Signals"=w104:waveform(dbl)[])  [unwired: 5 in, 1 out]
        n74 = disable-structure shown="Disabled" {
          disable-tunnel: [w162 w163] -> _
          disable-tunnel: [w161 _] -> w118
          frame Disabled {
            n75 = call "parse_KH_string.vi"() -> ("Measurement type"=w161:i32[], "Gain"=w162:dbl[])  [unwired: 10 in]
          }
          frame Enabled {
            n76 = Initialize Array(1.0) -> (w163:dbl[])  [unwired: 1 in]
          }
        }
        "Measure?" <- w118
        n77 = case shown="True" "measure offset" {
          tunnel: w104 -> [_ w150]
          frame False {
          }
          frame True {
            n78 = for {
              tunnel: [w154] -> w151 mode=indexing
              tunnel: w150 -> [w153] mode=indexing
              n79 = Unbundle By Name(w153) -> ("Y"=w152:dbl[])
              n80 = call-poly <vilib>:"Mean.vi"("X"=w152) -> ("mean"=w154:dbl)  [unwired: 1 out]
            }
            "offsets" <- w151
          }
        }
        n81 = local read "offsets"() -> (w105:dbl[])
        n82 = for {
          tunnel: w104 -> [w157] mode=indexing
          tunnel: [w156] -> w100 mode=indexing
          tunnel: w105 -> [w155] mode=indexing
          n83 = Subtract(x=w157, y=w155) -> (x-y=w156:waveform(dbl))
        }
        "Waveform Graph" <- w100
        n84 = for {
          tunnel: w100 -> [w160] mode=indexing
          tunnel: [w159] -> w102 mode=indexing
          tunnel: "Gain" -> [w158] mode=indexing
          n85 = Divide(x=w160, y=w158) -> (x/y=w159:waveform(dbl))
        }
        n86 = for {
          tunnel: "decimating factor 2" -> [w168]
          tunnel: w100 -> [w167] mode=indexing
          tunnel: [w166] -> _ mode=indexing
          n87 = call-poly <vilib>:"Decimate (single shot).vi"("averaging"=FALSE, "decimating factor"=w168, "X"=w167) -> ("Decimated Array"=w166:dbl[])  [unwired: 7 in, 1 out]
        }
        n88 = for {
          tunnel: w102 -> [w149] mode=indexing
          tunnel: [w148] -> w103 mode=indexing
          n89 = Unbundle By Name(w149) -> ("Y"=w148:dbl[])
        }
        n90 = Less?(x=w115, y=10) -> (x < y?=w107:bool)
        n91 = Or(x="zero offset", y=w107) -> (x .or. y?=w106:bool)
        n92 = Select(t=w110, s=w106, f=w113) -> (s? t:f=w112:dbl[])
        n93 = local write "offsets"(w112) -> ()
        n94 = local read "Sampling information"() -> (w143:cluster{"Fs":dbl, "#s":dbl}[])
        n95 = global read "Lock-in Globles Multiple Inputs and Outputs used with FGV.vi" "Multiplication factor"() -> (w142:dbl)
        n96 = call "Input Signals FGV.vi"("Function"=enum16{"write", "read"}."write", "Input Signals"=w103) -> ()  [unwired: 4 in, 2 out]
        n97 = local read "AO Task"() -> (w136:refnum<k21>[])
        n98 = call "Input Signals Waveform FGV.vi"("Function"=enum16{"write", "read"}."write", "input signal"=w102) -> ()  [unwired: 4 in, 2 out]
        n99 = case shown="True" TRUE {
          tunnel: w143 -> [_ w176]
          tunnel: w142 -> [_ w174]
          tunnel: w136 -> [_ w175]
          tunnel: [w169 w172] -> w126
          tunnel: w124 -> [_ w173]
          frame False {
            n100 = call "Output FGV.vi"("Function"=enum16{"write", "read"}."read") -> ("Output"=w169:waveform(dbl)[][])  [unwired: 5 in, 1 out]
          }
          frame True {
            n101 = call "Get Write Data.vi"("Multiplication Factor"=w174, "Sampling information 2"=w176, "AO Task"=w175, "OSC Configuration"=w173) -> ("Data"=w172:waveform(dbl)[][])  [unwired: 7 in]
            n102 = call "Output FGV.vi"("Function"=enum16{"write", "read"}."write", "Output"=w172) -> ()  [unwired: 4 in, 2 out]
          }
        }
        n103 = Get Date/Time In Seconds() -> (seconds since 1Jan1904=w144:timestamp)
        n104 = Index Array(array=w136) -> (element #1=w135:refnum<k21>, element #2=w134:refnum<k21>, element #3=w133:refnum<k21>, element #4=w132:refnum<k21>)  [unwired: 4 in]
        n105 = global write "Lock-in Globles Multiple Inputs and Outputs used with FGV.vi" "timestamp"(w144) -> ()
        n106 = Index Array(array=w126) -> (element #1=w131:waveform(dbl)[], element #2=w130:waveform(dbl)[], element #3=w129:waveform(dbl)[], element #4=w128:waveform(dbl)[])  [unwired: 8 in]
        n107 = call-poly <vilib>:"DAQmx Write.vi"("task/channels in"=w135, "data"=w131) -> ()  [unwired: 11 in, 3 out]
        n108 = call-poly <vilib>:"DAQmx Write.vi"("task/channels in"=w134, "data"=w130) -> ()  [unwired: 11 in, 3 out]
        n109 = call-poly <vilib>:"DAQmx Write.vi"("task/channels in"=w133, "data"=w129) -> ()  [unwired: 11 in, 3 out]
        n110 = call-poly <vilib>:"DAQmx Write.vi"("task/channels in"=w132, "data"=w128) -> ()  [unwired: 11 in, 3 out]
      }
      frame 3 {
        (unwired) TRUE ("Calculate REF?")
        # "make only one reference"
        # "OR statement goes here:\nlook for changes to OSC"
        # "The code to the right sends the lockin analysis results to one graph in each tab, then sends the current value of the current tab to Display 1 and Display 2"
        # "This code does lockin analysis of the data that was read, and then displays the results.  The result is multiplied by the gain for each element of the results."
        n111 = local read "reset lockin & averaging"() -> (w225:bool)
        n112 = local read "Remote"() -> (w270:bool)
        n113 = case shown="True" w270 {
          tunnel: [w328 w329] -> w267
          frame False {
            n114 = local read "OSC Configuration"() -> (w328:T4)
          }
          frame True {
            n115 = call "OSC Configuration FGV.vi"("Function"=enum16{"write", "read"}."read") -> ("OSC Configuration"=w329:T4)  [unwired: 5 in, 1 out]
          }
        }
        n116 = local read "Sampling information"() -> (w252:cluster{"Fs":dbl, "#s":dbl}[])
        n117 = local read "AI Block Size"() -> (w269:i32)
        n118 = local read "phase log"() -> (w266:dbl[])
        n119 = local read "AI Rate"() -> (w268:dbl)
        n120 = Initialize Array(0.0, 8 ("dimension size")) -> (w228:dbl[])
        n121 = Select(t=w228, s=w225, f=w229) -> (s? t:f=w226:dbl[])
        n122 = Select(t=w228, s=w225, f=w230) -> (s? t:f=w227:dbl[])
        n123 = Less?(x=w241, y=10) -> (x < y?=w242:bool)
        n124 = Array Size(array=w222) -> (size(s)=w237:i32)
        n125 = Index Array(array=w252) -> (element=w248:cluster{"Fs":dbl, "#s":dbl})  [unwired: 1 in]
        n126 = call "Get Reference for Demodulation.vi"("AI Block Size"=w269, "# channels"=w237, "Calculate REF?"=w242, "AI Rate"=w268, "OSC Configuration"=w267, "Phase&Tc"="Phase&Tc", "phase log"=w266, "Results"=w251) -> ("REF"=w255:T13, "Phase Log Out"=w265:dbl[], "Phase&Tc Out"=w264:T5)  [unwired: 5 in]
        n127 = Index Array(array=w255) -> (element=w254:T14)  [unwired: 1 in]
        n128 = Unbundle By Name(w254) -> ("Ref X"=w221:dbl[], "Ref Y"=w253:dbl[])
        n129 = Unbundle By Name(w248) -> ("Fs"=w249:dbl, "#s"=w246:dbl)
        n130 = node(w249) -> (w247:dbl[unit])
        n131 = local write "Phase&Tc"(w264) -> ()
        n132 = local write "phase log"(w265) -> ()
        n133 = Bundle By Name(cluster=cluster{"Fs":dbl[unit], "#S":i32} {"Fs"=55872.0, "#S"=8192} ("Sampling Info"), "Fs"=w247, "#S"=w246) -> (w223:cluster{"Fs":dbl[unit], "#S":i32})
        n134 = for {
          tunnel: w222 -> [w311] mode=indexing
          tunnel: w221 -> [w310]
          tunnel: w253 -> [w309]
          tunnel: "Filter Type" -> [w299]
          tunnel: "Cutoff Freq" -> [w300]
          tunnel: w223 -> [w301]
          tunnel: [w308] -> w235 mode=indexing
          tunnel: [w307] -> w234 mode=indexing
          tunnel: w227 -> [w302] mode=indexing
          tunnel: w226 -> [w306] mode=indexing
          tunnel: "Rolling Avg Parameters" -> [w305]
          tunnel: [w304] -> _ mode=indexing
          tunnel: [w303] -> _ mode=indexing
          tunnel: w241 -> [w296]
          i -> [w298]
          n135 = global read "Lock-in Globles Multiple Inputs and Outputs used with FGV.vi" "Reset Lockin"() -> (w293:bool)
          n136 = Less?(x=w296, y=10) -> (x < y?=w294:bool)
          n137 = Compound Arithmetic op=OR(w293, w294, "reset lockin & averaging") -> (w295:bool)
          n138 = case shown="0, Default" w298 {
            tunnel: w311 -> [w327]
            tunnel: w310 -> [w326]
            tunnel: w309 -> [w325]
            tunnel: [w324] -> w308
            tunnel: [w323] -> w307
            tunnel: w306 -> [w322]
            tunnel: w305 -> [w313]
            tunnel: [w321] -> w304
            tunnel: [w320] -> w303
            tunnel: w302 -> [w319]
            tunnel: w301 -> [w316]
            tunnel: w300 -> [w315]
            tunnel: w299 -> [w314]
            tunnel: w295 -> [w312]
            frame 0, Default {
              n139 = call "Patrick-UTiLIA-Lock.vi"("Reset Filter?"=w312, "Sampling Info"=w316, "Cutoff Freq"=w315, "Filter Type"=w314, "Unit Reference"=w325, "Noisy Signal"=w327) -> ("Locked Signal"=w318:dbl[])  [unwired: 1 out]
              n140 = call "Patrick-UTiLIA-Lock.vi"("Reset Filter?"=w312, "Sampling Info"=w316, "Cutoff Freq"=w315, "Filter Type"=w314, "Unit Reference"=w326, "Noisy Signal"=w327) -> ("Locked Signal"=w317:dbl[])  [unwired: 1 out]
              n141 = call "Patrick-UTiLIA-RollingAverage.vi"("Restart Avg"=w312, "Current Average"=w322, "Rolling Avg Parameters"=w313, "Signal to Average"=w317) -> ("Long-term Average"=w323:dbl, "Chunk Average"=w321:dbl)  [unwired: 3 out]
              n142 = call "Patrick-UTiLIA-RollingAverage.vi"("Restart Avg"=w312, "Current Average"=w319, "Rolling Avg Parameters"=w313, "Signal to Average"=w318) -> ("Long-term Average"=w324:dbl, "Chunk Average"=w320:dbl)  [unwired: 3 out]
            }
          }
        }
        n143 = global read "Lock-in Globles Multiple Inputs and Outputs used with FGV.vi" "Stop Lockin"() -> (w276:bool)
        n144 = local read "Measure?"() -> (w236:u16[])
        n145 = case shown="\"FFT\"" "Tab Control" {
          tunnel: w222 -> [_ w281]
          frame "Input signals", Default {
          }
          frame "FFT" {
            n146 = global read "Lock-in Globles Multiple Inputs and Outputs used with FGV.vi" "Reset Lockin"() -> (w285:bool)
            n147 = call-poly <vilib>:"FFT Power Spectrum and PSD.vi"("averaging parameters"="averaging parameters", "restart averaging (F)"=w285, "dB On (F)"="dB On (F)", "window"="window", "time signals"=w281) -> ("Power Spectrum / PSD"=→"Waveform Graph 2":cluster{"f0":dbl, "df":dbl, "magnitude":dbl[]}[])  [unwired: 3 in, 3 out]
          }
        }
        n148 = global read "Lock-in Globles Multiple Inputs and Outputs used with FGV.vi" "Reset Lockin"() -> (w258:bool)
        n149 = Or(x=w276, y="stop") -> (x .or. y?=w274:bool)
        n150 = Decrement(x="Input Signals") -> (x-1=w260:i16)
        n151 = Select(t=4.0 ("f"), s=w274, f=2.0) -> (s? t:f=w273:dbl)
        n152 = for {
          tunnel: w234 -> [w286] mode=indexing
          tunnel: w235 -> [w288] mode=indexing
          tunnel: [w287] -> w224 mode=indexing
          n153 = Re/Im To Polar(2:w288, 3:w286) -> (0:w291:dbl, 1:w289:dbl)
          n154 = expression code="x * 180/pi"(w291) -> (w290:dbl)
          n155 = Build Array(w286, w288, w289, w290) -> (w287:dbl[])
        }
        "Results (X, Y, R, Theta)" <- w224
        n156 = call "Display.vi"("Results"=w224, "Display"="Display", "Lock-in #"=w260, "Amplifier Settings"=w236) -> ("Display 1"=→"Display 1":string, "Display 2"=→"Display 2":string, "Array"=→"Display X (or R) A":dbl[], "Array 2"=→"Display Y (or Theta) A":dbl[])  [unwired: 3 in]
        n157 = Select(t=5.0, s=w258, f=w273) -> (s? t:f=w271:dbl)
        n158 = call "Results FGV.vi"("Function"=enum16{"write", "read"}."write", "Input Signals"=w224) -> ()  [unwired: 4 in, 2 out]
      }
      frame 4 {
        # "This code stops the AI/AO Tasks, erases them, and ends program execution."
        n159 = local read "AO Task"() -> (w339:refnum<k21>[])
        n160 = local read "AI task"() -> (w341:refnum<k21>[])
        n161 = flat-sequence {
          tunnel: w341 -> [w353]
          tunnel: [w352] -> w340
          tunnel: w339 -> [w352]
          tunnel: [w351] -> w338
          tunnel: w340 -> [w359]
          tunnel: w338 -> [w358]
          tunnel: [w358] -> w337
          tunnel: [w357] -> w336
          frame #0 {
            n162 = for {
              tunnel: w353 -> [w356] mode=indexing
              tunnel: [w354] -> w351 mode=indexing
              n163 = call <vilib>:"DAQmx Stop Task.vi"("task/channels in"=w356) -> ("task out"=w354:refnum<k21>)  [unwired: 13 in, 1 out]
              n164 = Wait (ms)(milliseconds to wait=u32 50) -> ()  [unwired: 1 out]
            }
          }
          frame #1 {
            n165 = for {
              tunnel: w359 -> [w362] mode=indexing
              tunnel: [w360] -> w357 mode=indexing
              n166 = call <vilib>:"DAQmx Stop Task.vi"("task/channels in"=w362) -> ("task out"=w360:refnum<k21>)  [unwired: 13 in, 1 out]
              n167 = Wait (ms)(milliseconds to wait=u32 50) -> ()  [unwired: 1 out]
            }
          }
        }
        n168 = flat-sequence {
          tunnel: w337 -> [w345]
          tunnel: w336 -> [w344]
          tunnel: [w344] -> w335
          tunnel: w335 -> [w348]
          frame #0 {
            n169 = for {
              tunnel: w345 -> [w347] mode=indexing
              n170 = Wait (ms)(milliseconds to wait=u32 50) -> ()  [unwired: 1 out]
              n171 = call <vilib>:"DAQmx Clear Task.vi"("task in"=w347) -> ()  [unwired: 14 in, 1 out]
            }
          }
          frame #1 {
            n172 = for {
              tunnel: w348 -> [w350] mode=indexing
              n173 = call <vilib>:"DAQmx Clear Task.vi"("task in"=w350) -> ()  [unwired: 14 in, 1 out]
              n174 = Wait (ms)(milliseconds to wait=u32 50) -> ()  [unwired: 1 out]
            }
          }
        }
      }
      frame 5 {
        # "This code stops AI/AO tasks, deletes them, and restarts program execution."
        n175 = local read "AO Task"() -> (w370:refnum<k21>[])
        n176 = local read "AI task"() -> (w371:refnum<k21>[])
        n177 = flat-sequence {
          tunnel: w371 -> [w378]
          tunnel: [w377] -> w373
          tunnel: w370 -> [w377]
          tunnel: [w376] -> w372
          tunnel: w373 -> [w384]
          tunnel: w372 -> [w383]
          tunnel: [w383] -> w369
          tunnel: [w382] -> w368
          tunnel: w369 -> [w388]
          tunnel: w368 -> [w389]
          tunnel: [w389] -> w367
          tunnel: w367 -> [w392]
          frame #0 {
            n178 = for {
              tunnel: w378 -> [w381] mode=indexing
              tunnel: [w379] -> w376 mode=indexing
              n179 = Wait (ms)(milliseconds to wait=u32 50) -> ()  [unwired: 1 out]
              n180 = call <vilib>:"DAQmx Stop Task.vi"("task/channels in"=w381) -> ("task out"=w379:refnum<k21>)  [unwired: 13 in, 1 out]
            }
          }
          frame #1 {
            n181 = for {
              tunnel: w384 -> [w387] mode=indexing
              tunnel: [w385] -> w382 mode=indexing
              n182 = Wait (ms)(milliseconds to wait=u32 50) -> ()  [unwired: 1 out]
              n183 = call <vilib>:"DAQmx Stop Task.vi"("task/channels in"=w387) -> ("task out"=w385:refnum<k21>)  [unwired: 13 in, 1 out]
            }
          }
          frame #2 {
            n184 = for {
              tunnel: w388 -> [w391] mode=indexing
              n185 = call <vilib>:"DAQmx Clear Task.vi"("task in"=w391) -> ()  [unwired: 14 in, 1 out]
              n186 = Wait (ms)(milliseconds to wait=u32 50) -> ()  [unwired: 1 out]
            }
          }
          frame #3 {
            n187 = for {
              tunnel: w392 -> [w394] mode=indexing
              n188 = call <vilib>:"DAQmx Clear Task.vi"("task in"=w394) -> ()  [unwired: 14 in, 1 out]
              n189 = Wait (ms)(milliseconds to wait=u32 50) -> ()  [unwired: 1 out]
            }
          }
        }
      }
    }
    "Numeric" <- w38
  }
  n190 = disable-structure shown="Enabled" {
    disable-tunnel: "Stream to disk?" -> [w395 _]
    frame Disabled {
      n191 = case shown="True" w395 {
        frame False {
        }
        frame True {
          w404 = FALSE ("averaging")
          n192 = Index Array() -> ()  [unwired: 9 in, 4 out]
          n193 = call-poly <vilib>:"Decimate (single shot).vi"("averaging"=w404, "decimating factor"="decimating factor") -> ("Decimated Array"=w403:dbl[])  [unwired: 8 in, 1 out]
          n194 = call-poly <vilib>:"Decimate (single shot).vi"("averaging"=w404, "decimating factor"="decimating factor") -> ("Decimated Array"=w402:dbl[])  [unwired: 8 in, 1 out]
          n195 = call-poly <vilib>:"Decimate (single shot).vi"("averaging"=w404, "decimating factor"="decimating factor") -> ("Decimated Array"=w401:dbl[])  [unwired: 8 in, 1 out]
          n196 = call <userlib>:"Read PPMS T and B.vi"() -> ("Field"=w398:dbl, "Temperature"=w399:dbl, "Time"=w400:dbl)  [unwired: 3 in]
          n197 = Build Array(w403, w402, w401) -> (w397:dbl[][])
          n198 = call "Stream_lock_in_data.vi"("Input signal 2"=w397, "decimating factor"="decimating factor", "Field"=w398, "Temperature"=w399, "Time"=w400) -> ()  [unwired: 4 in]
        }
      }
    }
    frame Enabled {
    }
  }
